vi "Launcher.vi"   [LabVIEW 2025]
uses:
  UI VISA Terminal.lvclass
  C:/Program Files/National Instruments/LabVIEW 2025/vi.lib/ActorFramework/Actor/Actor.lvclass
  a1887efa-5063-44be-9f6c-3d0f707cfce3.vi
  <vilib>/ActorFramework/Actor/Actor.lvclass
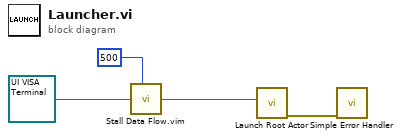
[diagram p0: block diagram]
diagram:
  n1 = call "Stall Data Flow.vim"("value in"=refnum<class "UI VISA Terminal.lvclass"> refnum ("UI VISA Terminal.lvlib:UI VISA Terminal.lvclass"), "milliseconds to wait"=u32 500) -> ("value out"=w2:refnum<class "UI VISA Terminal.lvclass">)  [unwired: 1 out]
  n2 = call <vilib>:"Launch Root Actor.vi"("Actor"=w2) -> ("error out"=w3:errorcluster)  [unwired: 9 in, 1 out]
  n3 = call <vilib>:"Simple Error Handler.vi"("error in (no error)"=w3) -> ()  [unwired: 4 in, 5 out]
